vi "Test Instrument Remote Client.vi"() -> ()   [LabVIEW 2019]
uses:
  lvsrc/Templates/Instrument.Template/Instrument.Template.lvclass
  C:/Users/patrick/Documents/GitHub/Instrument-Framework/lvsrc/SMOs/Instrument/Instrument.lvclass
  lvsrc/SMOs/Instrument/Instrument.lvclass
panel:
  out "Waveform Chart":cluster{dbl, dbl, dbl}(graph)
  in  "stop":bool
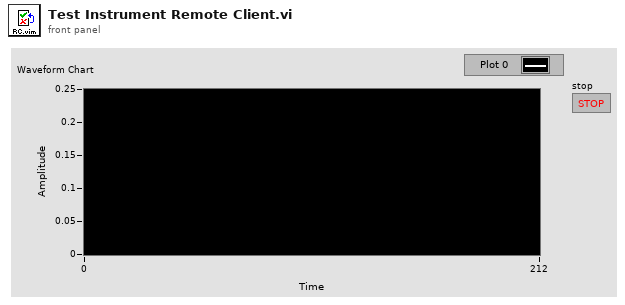
[diagram p1: front panel]
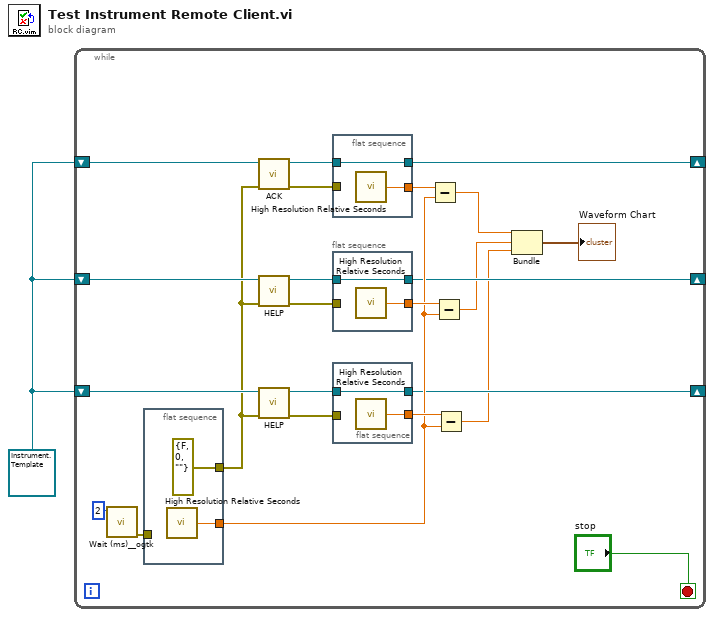
[diagram p0: block diagram]
diagram:
  w1 = refnum<class "Instrument.Template.lvclass"> refnum ("Instrument.Template.lvclass")
  n1 = while {
    shift-right: [w8] -> _
    shift-left: w1 -> [w18]
    shift-right: [w9] -> _
    shift-left: w1 -> [w21]
    shift-right: [w10] -> _
    shift-left: w1 -> [w15]
    stop <- "stop" stop-if-true
    n2 = call <userlib>:"Wait (ms)__ogtk.vi"("milliseconds to wait"=u32 2) -> ("error out"=w3:errorcluster)  [unwired: 9 in, 1 out]
    n3 = flat-sequence {
      tunnel: [errorcluster {"status"=FALSE, "code"=0, "source"=""} ("error in (no error)")] -> w12
      tunnel: [w32] -> w22
      tunnel: w3 -> [_]
      frame #0 {
        n4 = call <vilib>:"High Resolution Relative Seconds.vi"() -> ("relative seconds"=w32:dbl)
      }
    }
    n5 = call "ACK.vi"("error in (no error)"=w12, "Instrument in"=w18) -> ("error out"=w16:errorcluster, "Instrument out"=w17:refnum<class "Instrument.Template.lvclass">)  [unwired: 7 in, 1 out]
    n6 = call "HELP.vi"("error in (no error)"=w12, "Instrument in"=w21) -> ("error out"=w19:errorcluster, "Instrument out"=w20:refnum<class "Instrument.Template.lvclass">)  [unwired: 7 in, 1 out]
    n7 = call "HELP.vi"("error in (no error)"=w12, "Instrument in"=w15) -> ("error out"=w13:errorcluster, "Instrument out"=w14:refnum<class "Instrument.Template.lvclass">)  [unwired: 7 in, 1 out]
    n8 = flat-sequence {
      tunnel: w16 -> [_]
      tunnel: [w31] -> w23
      tunnel: w17 -> [w30]
      tunnel: [w30] -> w8
      frame #0 {
        n9 = call <vilib>:"High Resolution Relative Seconds.vi"() -> ("relative seconds"=w31:dbl)
      }
    }
    n10 = flat-sequence {
      tunnel: w19 -> [_]
      tunnel: [w29] -> w24
      tunnel: w20 -> [w28]
      tunnel: [w28] -> w9
      frame #0 {
        n11 = call <vilib>:"High Resolution Relative Seconds.vi"() -> ("relative seconds"=w29:dbl)
      }
    }
    n12 = flat-sequence {
      tunnel: w13 -> [_]
      tunnel: [w27] -> w25
      tunnel: w14 -> [w26]
      tunnel: [w26] -> w10
      frame #0 {
        n13 = call <vilib>:"High Resolution Relative Seconds.vi"() -> ("relative seconds"=w27:dbl)
      }
    }
    n14 = Subtract(x=w23, y=w22) -> (x-y=w6:dbl)
    n15 = Subtract(x=w24, y=w22) -> (x-y=w7:dbl)
    n16 = Subtract(x=w25, y=w22) -> (x-y=w5:dbl)
    n17 = Bundle(w6, w7, w5) -> (→"Waveform Chart":cluster{dbl, dbl, dbl})  [unwired: 1 in]
  }
